vi "unimplemented_refs.vi"() -> ()   [LabVIEW 2021]
panel:
  in  "References":T1
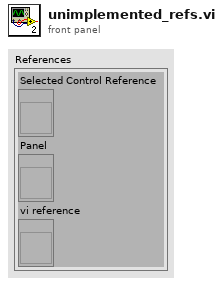
[diagram p1: front panel]
types:
  T1 = cluster{"Selected Control Reference":refnum<vi>, "Panel":refnum<vi>, "vi reference":refnum<vi>}
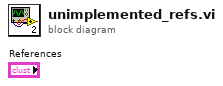
[diagram p0: block diagram]
diagram:
